vi "VI Server_GetControlRange.vi"(6 "Default.Maximum":dbl=3000.0 format="%#_15g", 7 "Default.Minimum":dbl format="%#_15g", 8 "error in (no error)":errorcluster, 9 "ControlReference":refnum<vi>) -> (0 "error out":errorcluster, 4 "Data Range":T1)   [LabVIEW 2020, in "VI Server Toolkit LV2013.lvlib"]
doc: "Returns the range of numeric control specified by its generic reference."
uses:
  VI Server Toolkit LV2013.lvlib
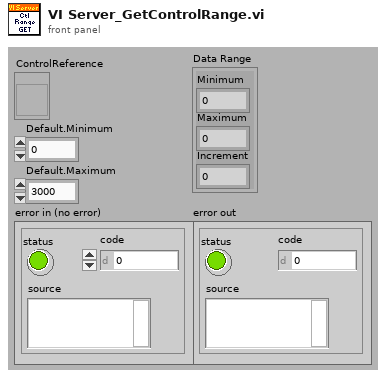
[diagram p1: front panel]
types:
  T1 = cluster{"Minimum":dbl, "Maximum":dbl, "Increment":dbl}
  T2 = typedef "LVMinMaxIncTypeDef.ctl" = cluster{"Minimum":dbl, "Maximum":dbl, "Increment":dbl}
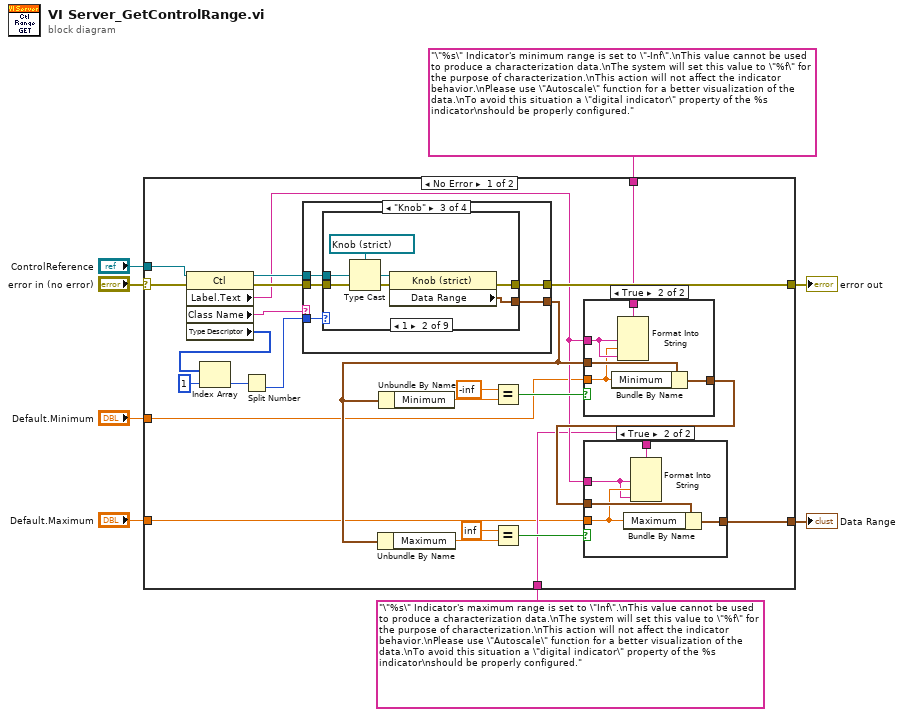
[diagram p0: block diagram]
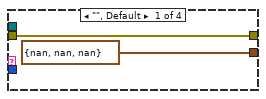
[diagram p4: hidden frame]
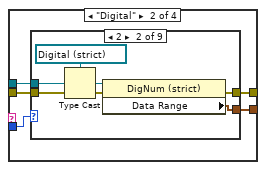
[diagram p5: hidden frame]
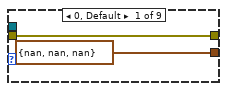
[diagram p6: hidden frame]
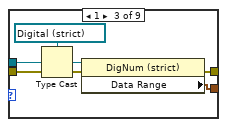
[diagram p7: hidden frame]
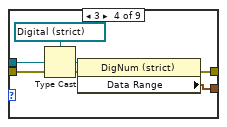
[diagram p8: hidden frame]
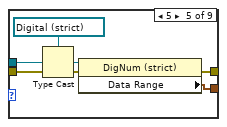
[diagram p9: hidden frame]
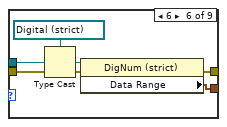
[diagram p10: hidden frame]
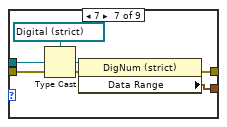
[diagram p11: hidden frame]
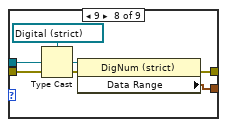
[diagram p12: hidden frame]
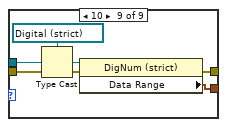
[diagram p13: hidden frame]
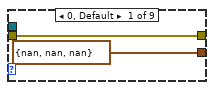
[diagram p14: hidden frame]
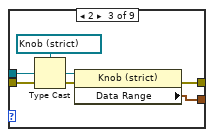
[diagram p15: hidden frame]
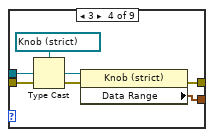
[diagram p16: hidden frame]
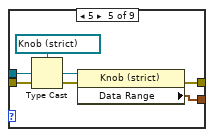
[diagram p17: hidden frame]
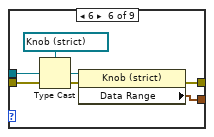
[diagram p18: hidden frame]
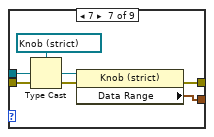
[diagram p19: hidden frame]
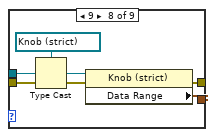
[diagram p20: hidden frame]
diagram:
  n1 = case shown="No Error" "error in (no error)" {
    selector: "error in (no error)" -> [w24 w212]
    tunnel: [w32 w212] -> w8
    tunnel: "ControlReference" -> [w31 _]
    tunnel: "\"%s\" Indicator's minimum range is set to \"-Inf\".\nThis value cannot be used to produce a characterization data.\nThe system will set this value to \"%f\" for the purpose of characterization.\nThis action will not affect the indicator behavior.\nPlease use \"Autoscale\" function for a better visualization of the data.\nTo avoid this situation a \"digital indicator\" property of the %s indicator\nshould be properly configured." ("format string") -> [w19 _]
    tunnel: "\"%s\" Indicator's maximum range is set to \"Inf\".\nThis value cannot be used to produce a characterization data.\nThe system will set this value to \"%f\" for the purpose of characterization.\nThis action will not affect the indicator behavior.\nPlease use \"Autoscale\" function for a better visualization of the data.\nTo avoid this situation a \"digital indicator\" property of the %s indicator\nshould be properly configured." ("format string") -> [w12 _]
    tunnel: [w11 T1 {"Minimum"=nan, "Maximum"=nan, "Increment"=nan} ("Data Range")] -> w4
    tunnel: "Default.Minimum" -> [w10 _]
    tunnel: "Default.Maximum" -> [w9 _]
    frame No Error {
      n2 = property class="Ctl"(reference=w31, error in=w24) -> (reference out=w30:refnum<vi>, error out=w28:errorcluster, "Label.Text"=w13:string, "Class Name"=w20:string, "Type Descriptor"=w27:i16[])
      n3 = Index Array(array=w27, index=1) -> (element=w25:i16)
      n4 = Split Number(x=w25) -> (lo(x)=w29:u8)  [unwired: 1 out]
      n5 = case shown="\"Knob\"" w20 {
        tunnel: w29 -> [_ w51 w106 w158]
        tunnel: w30 -> [_ w49 w104 w160]
        tunnel: w28 -> [w46 w50 w105 w161]
        tunnel: [w46 w48 w103 w159] -> w32
        tunnel: [T1 {"Minimum"=nan, "Maximum"=nan, "Increment"=nan} ("Data Range") w47 w102 w157] -> w16
        frame "", Default {
        }
        frame "Digital" {
          n6 = case shown="2" w51 {
            tunnel: w50 -> [w53 w59 w65 w71 w77 w83 w89 w95 w101]
            tunnel: w49 -> [_ w58 w64 w70 w76 w82 w88 w94 w100]
            tunnel: [w53 w56 w62 w68 w74 w79 w86 w92 w98] -> w48
            tunnel: [T1 {"Minimum"=nan, "Maximum"=nan, "Increment"=nan} ("Data Range") w54 w60 w66 w72 w78 w84 w90 w96] -> w47
            frame 0, Default {
            }
            frame 2 {
              n7 = Type Cast(type=refnum<vi> refnum ("Numeric"), x=w58) -> (*(type *) &x=w57:refnum<vi>)
              n8 = property class="DigNum (strict)"(reference=w57, error in=w59) -> (error out=w56:errorcluster, "Data Range"=w54:T2)  [unwired: 1 out]
            }
            frame 1 {
              n9 = Type Cast(type=refnum<vi> refnum ("Numeric"), x=w64) -> (*(type *) &x=w63:refnum<vi>)
              n10 = property class="DigNum (strict)"(reference=w63, error in=w65) -> (error out=w62:errorcluster, "Data Range"=w60:T2)  [unwired: 1 out]
            }
            frame 3 {
              n11 = Type Cast(type=refnum<vi> refnum ("Numeric"), x=w70) -> (*(type *) &x=w69:refnum<vi>)
              n12 = property class="DigNum (strict)"(reference=w69, error in=w71) -> (error out=w68:errorcluster, "Data Range"=w66:T2)  [unwired: 1 out]
            }
            frame 5 {
              n13 = Type Cast(type=refnum<vi> refnum ("Numeric"), x=w76) -> (*(type *) &x=w75:refnum<vi>)
              n14 = property class="DigNum (strict)"(reference=w75, error in=w77) -> (error out=w74:errorcluster, "Data Range"=w72:T2)  [unwired: 1 out]
            }
            frame 6 {
              n15 = Type Cast(type=refnum<vi> refnum ("Numeric"), x=w82) -> (*(type *) &x=w80:refnum<vi>)
              n16 = property class="DigNum (strict)"(reference=w80, error in=w83) -> (error out=w79:errorcluster, "Data Range"=w78:T2)  [unwired: 1 out]
            }
            frame 7 {
              n17 = Type Cast(type=refnum<vi> refnum ("Numeric"), x=w88) -> (*(type *) &x=w87:refnum<vi>)
              n18 = property class="DigNum (strict)"(reference=w87, error in=w89) -> (error out=w86:errorcluster, "Data Range"=w84:T2)  [unwired: 1 out]
            }
            frame 9 {
              n19 = Type Cast(type=refnum<vi> refnum ("Numeric"), x=w94) -> (*(type *) &x=w93:refnum<vi>)
              n20 = property class="DigNum (strict)"(reference=w93, error in=w95) -> (error out=w92:errorcluster, "Data Range"=w90:T2)  [unwired: 1 out]
            }
            frame 10 {
              n21 = Type Cast(type=refnum<vi> refnum ("Numeric"), x=w100) -> (*(type *) &x=w99:refnum<vi>)
              n22 = property class="DigNum (strict)"(reference=w99, error in=w101) -> (error out=w98:errorcluster, "Data Range"=w96:T2)  [unwired: 1 out]
            }
          }
        }
        frame "Knob" {
          n23 = case shown="1" w106 {
            tunnel: w105 -> [w108 w114 w117 w126 w132 w138 w144 w147 w153]
            tunnel: w104 -> [_ w113 w120 w125 w131 w137 w143 w150 w156]
            tunnel: [w108 w110 w119 w122 w128 w134 w140 w149 w155] -> w103
            tunnel: [T1 {"Minimum"=nan, "Maximum"=nan, "Increment"=nan} ("Data Range") w109 w115 w121 w127 w133 w139 w145 w151] -> w102
            frame 0, Default {
            }
            frame 1 {
              n24 = Type Cast(type=refnum<vi> refnum ("Knob"), x=w113) -> (*(type *) &x=w111:refnum<vi>)
              n25 = property class="Knob (strict)"(reference=w111, error in=w114) -> (error out=w110:errorcluster, "Data Range"=w109:T2)  [unwired: 1 out]
            }
            frame 2 {
              n26 = Type Cast(type=refnum<vi> refnum ("Knob"), x=w120) -> (*(type *) &x=w116:refnum<vi>)
              n27 = property class="Knob (strict)"(reference=w116, error in=w117) -> (error out=w119:errorcluster, "Data Range"=w115:T2)  [unwired: 1 out]
            }
            frame 3 {
              n28 = Type Cast(type=refnum<vi> refnum ("Knob"), x=w125) -> (*(type *) &x=w124:refnum<vi>)
              n29 = property class="Knob (strict)"(reference=w124, error in=w126) -> (error out=w122:errorcluster, "Data Range"=w121:T2)  [unwired: 1 out]
            }
            frame 5 {
              n30 = Type Cast(type=refnum<vi> refnum ("Knob"), x=w131) -> (*(type *) &x=w130:refnum<vi>)
              n31 = property class="Knob (strict)"(reference=w130, error in=w132) -> (error out=w128:errorcluster, "Data Range"=w127:T2)  [unwired: 1 out]
            }
            frame 6 {
              n32 = Type Cast(type=refnum<vi> refnum ("Knob"), x=w137) -> (*(type *) &x=w136:refnum<vi>)
              n33 = property class="Knob (strict)"(reference=w136, error in=w138) -> (error out=w134:errorcluster, "Data Range"=w133:T2)  [unwired: 1 out]
            }
            frame 7 {
              n34 = Type Cast(type=refnum<vi> refnum ("Knob"), x=w143) -> (*(type *) &x=w142:refnum<vi>)
              n35 = property class="Knob (strict)"(reference=w142, error in=w144) -> (error out=w140:errorcluster, "Data Range"=w139:T2)  [unwired: 1 out]
            }
            frame 9 {
              n36 = Type Cast(type=refnum<vi> refnum ("Knob"), x=w150) -> (*(type *) &x=w146:refnum<vi>)
              n37 = property class="Knob (strict)"(reference=w146, error in=w147) -> (error out=w149:errorcluster, "Data Range"=w145:T2)  [unwired: 1 out]
            }
            frame 10 {
              n38 = Type Cast(type=refnum<vi> refnum ("Knob"), x=w156) -> (*(type *) &x=w152:refnum<vi>)
              n39 = property class="Knob (strict)"(reference=w152, error in=w153) -> (error out=w155:errorcluster, "Data Range"=w151:T2)  [unwired: 1 out]
            }
          }
        }
        frame "Slide" {
          n40 = case shown="10" w158 {
            tunnel: w161 -> [w163 w165 w171 w177 w183 w189 w195 w201 w207]
            tunnel: w160 -> [_ w169 w175 w181 w187 w193 w199 w205 w211]
            tunnel: [w163 w167 w174 w180 w186 w192 w198 w204 w210] -> w159
            tunnel: [T1 {"Minimum"=nan, "Maximum"=nan, "Increment"=nan} ("Data Range") w166 w172 w178 w184 w190 w196 w202 w208] -> w157
            frame 0, Default {
            }
            frame 1 {
              n41 = Type Cast(type=refnum<vi> refnum ("Slide"), x=w169) -> (*(type *) &x=w164:refnum<vi>)
              n42 = property class="Slide (strict)"(reference=w164, error in=w165) -> (error out=w167:errorcluster, "Data Range"=w166:T2)  [unwired: 1 out]
            }
            frame 2 {
              n43 = Type Cast(type=refnum<vi> refnum ("Slide"), x=w175) -> (*(type *) &x=w170:refnum<vi>)
              n44 = property class="Slide (strict)"(reference=w170, error in=w171) -> (error out=w174:errorcluster, "Data Range"=w172:T2)  [unwired: 1 out]
            }
            frame 3 {
              n45 = Type Cast(type=refnum<vi> refnum ("Slide"), x=w181) -> (*(type *) &x=w176:refnum<vi>)
              n46 = property class="Slide (strict)"(reference=w176, error in=w177) -> (error out=w180:errorcluster, "Data Range"=w178:T2)  [unwired: 1 out]
            }
            frame 5 {
              n47 = Type Cast(type=refnum<vi> refnum ("Slide"), x=w187) -> (*(type *) &x=w182:refnum<vi>)
              n48 = property class="Slide (strict)"(reference=w182, error in=w183) -> (error out=w186:errorcluster, "Data Range"=w184:T2)  [unwired: 1 out]
            }
            frame 6 {
              n49 = Type Cast(type=refnum<vi> refnum ("Slide"), x=w193) -> (*(type *) &x=w188:refnum<vi>)
              n50 = property class="Slide (strict)"(reference=w188, error in=w189) -> (error out=w192:errorcluster, "Data Range"=w190:T2)  [unwired: 1 out]
            }
            frame 7 {
              n51 = Type Cast(type=refnum<vi> refnum ("Slide"), x=w199) -> (*(type *) &x=w194:refnum<vi>)
              n52 = property class="Slide (strict)"(reference=w194, error in=w195) -> (error out=w198:errorcluster, "Data Range"=w196:T2)  [unwired: 1 out]
            }
            frame 9 {
              n53 = Type Cast(type=refnum<vi> refnum ("Slide"), x=w205) -> (*(type *) &x=w200:refnum<vi>)
              n54 = property class="Slide (strict)"(reference=w200, error in=w201) -> (error out=w204:errorcluster, "Data Range"=w202:T2)  [unwired: 1 out]
            }
            frame 10 {
              n55 = Type Cast(type=refnum<vi> refnum ("Slide"), x=w211) -> (*(type *) &x=w206:refnum<vi>)
              n56 = property class="Slide (strict)"(reference=w206, error in=w207) -> (error out=w210:errorcluster, "Data Range"=w208:T2)  [unwired: 1 out]
            }
          }
        }
      }
      n57 = Unbundle By Name(w16) -> ("Maximum"=w18:dbl)
      n58 = Unbundle By Name(w16) -> ("Minimum"=w21:dbl)
      n59 = Equal?(x=-inf, y=w21) -> (x = y?=w22:bool)
      n60 = Equal?(x=inf, y=w18) -> (x = y?=w15:bool)
      n61 = case shown="True" w22 {
        tunnel: w16 -> [w39 w44]
        tunnel: w13 -> [_ w41]
        tunnel: w19 -> [_ w43]
        tunnel: [w39 w42] -> w14
        tunnel: w10 -> [_ w40]
        frame False {
        }
        frame True {
          n62 = Bundle By Name(cluster=w44, "Minimum"=w40) -> (w42:T2)
          n63 = Format Into String(format string=w43, w41, w40, w41) -> ()  [unwired: 2 in, 2 out]
        }
      }
      n64 = case shown="True" w15 {
        tunnel: w14 -> [w33 w38]
        tunnel: w13 -> [_ w34]
        tunnel: w12 -> [_ w37]
        tunnel: [w33 w36] -> w11
        tunnel: w9 -> [_ w35]
        frame False {
        }
        frame True {
          n65 = Bundle By Name(cluster=w38, "Maximum"=w35) -> (w36:T2)
          n66 = Format Into String(format string=w37, w34, w35, w34) -> ()  [unwired: 2 in, 2 out]
        }
      }
    }
    frame Error {
    }
  }
  "error out" <- w8
  "Data Range" <- w4
